vi "Read Filesystem Statistics.vi"(8 "error in":errorcluster, 10 "remote path":string, 11 "session in":refnum<class "Session.lvclass">) -> (0 "error out":errorcluster, 2 "filesystem statistics":refnum<class "Filesystem Statistics.lvclass">, 3 "session out":refnum<class "Session.lvclass">)   [LabVIEW 2020, in "NI_SFTP.lvlib"]
doc: "Returns information about the disk or filesystem that contains the specified path, including total space and free space. The server must support OpenSSH extensions."
uses:
  <vilib>/net/SFTP/NI_SFTP.lvlib
  <vilib>/net/SFTP/Session/Session.lvclass
  <vilib>/net/SFTP/Filesystem Statistics/Filesystem Statistics.lvclass
  <vilib>/net/SFTP/API/Support/Command/statvfs_openssh.com/statvfs_openssh.com.lvclass
  <vilib>/Utility/Deadline/NI_Deadline.lvlib
panel:
  in  "timeout (ms)":i32=30000
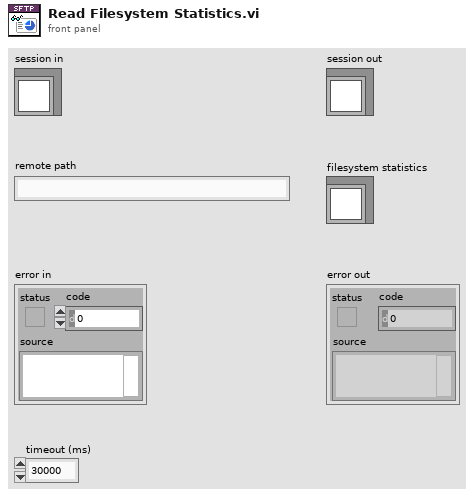
[diagram p1: front panel]
types:
  T1 = typedef "NI_Deadline.lvlib/Deadline.ctl" = cluster{"mode":T2, "deadline (ms)":u32}
  T2 = typedef "NI_Deadline.lvlib/Mode.ctl" = enum16{"Relative", "Use deadline", "Wait forever", "Nonblocking", "N/A"}
  T3 = typedef "NI_SFTP.lvlib/statvfs info.ctl" = cluster{"f_bsize":u64, "f_frsize":u64, "f_blocks":u64, "f_bfree":u64, "f_bavail":u64, "f_files":u64, "f_ffree":u64, "f_favail":u64, "f_fsid":u64, "f_flag":u64, "f_namemax":u64}
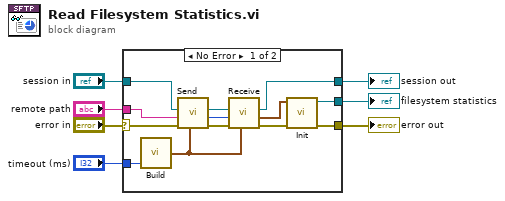
[diagram p0: block diagram]
diagram:
  n1 = case shown="No Error" "error in" {
    selector: "error in" -> [w20 w21]
    tunnel: "session in" -> [w11 w22]
    tunnel: "remote path" -> [w12 _]
    tunnel: [w8 w22] -> w1
    tunnel: [w16 w21] -> w4
    tunnel: [w15 _] -> w3
    tunnel: "timeout (ms)" -> [w14 _]
    frame No Error {
      n2 = call <vilib>:"Build.vi"("timeout (ms)"=w14) -> ("Deadline out"=w13:T1)  [unwired: 2 in]
      n3 = call <vilib>:"Send.vi"("Timeout"=w13, "error in (no error)"=w20, "path"=w12, "session in"=w11) -> ("error out"=w19:errorcluster, "request id"=w10:u32, "session out"=w18:refnum<class "Session.lvclass">)  [unwired: 4 in, 1 out]
      n4 = call <vilib>:"Receive.vi"("Timeout"=w13, "error in (no error)"=w19, "request id"=w10, "session in"=w18) -> ("error out"=w17:errorcluster, "statistics"=w9:T3, "session out"=w8:refnum<class "Session.lvclass">)  [unwired: 4 in, 1 out]
      n5 = call <vilib>:"Init.vi"("error in"=w17, "statvfs info"=w9) -> ("error out"=w16:errorcluster, "Filesystem Statistics out"=w15:refnum<class "Filesystem Statistics.lvclass">)  [unwired: 8 in]
    }
    frame Error {
    }
  }
  "error out" <- w4
  "session out" <- w1
  "filesystem statistics" <- w3
